vi "发送测试脚本.vi"(7 "Script Name":string="TSB_Script", 8 "错误输入":errorcluster, 11 "Script":string) -> (0 "错误输出":errorcluster)   [LabVIEW 2020]
uses:
  VISA 2601B.vi
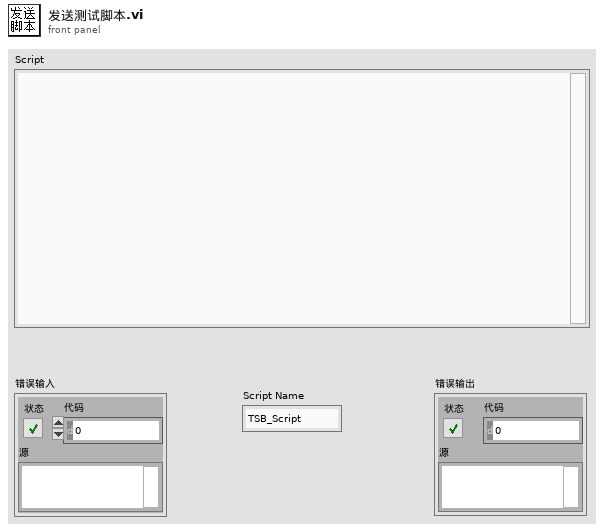
[diagram p1: front panel]
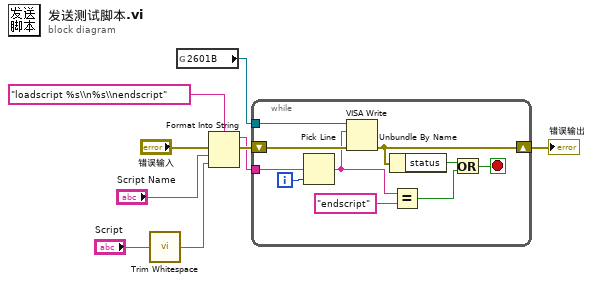
[diagram p0: block diagram]
diagram:
  n1 = call <vilib>:"Trim Whitespace.vi"("string"="Script") -> ("trimmed string"=w1:string)  [unwired: 1 in]
  n2 = global read "VISA 2601B.vi" "2601B"() -> (w3:refnum<visa-resource-name>)
  n3 = Format Into String(format string="loadscript %s\\n%s\\nendscript", error in="错误输入", "Script Name", w1) -> (resulting string=w2:string, error out=w4:errorcluster)  [unwired: 1 in]
  n4 = while {
    tunnel: w3 -> [w18]
    shift-right: [w12] -> w7
    shift-left: w4 -> [w19]
    tunnel: w2 -> [w16]
    i -> [w15]
    stop <- w10 stop-if-true
    n5 = Pick Line(multi-line string=w16, line index=w15) -> (output string=w11:string)  [unwired: 1 out]
    n6 = VISA Write(VISA resource name=w18, write buffer=w11, error in (no error)=w19) -> (error out=w12:errorcluster)  [unwired: 2 out]
    n7 = Unbundle By Name(w12) -> ("status"=w14:bool)
    n8 = Equal?(x=w11, y="endscript") -> (x = y?=w13:bool)
    n9 = Or(x=w14, y=w13) -> (x .or. y?=w10:bool)
  }
  "错误输出" <- w7
